vi "DAC Init Results.vi"(8 "error in":errorcluster, 9 "Log Details?":bool, 10 "tdms file":refnum<k34>, 11 "DAC FTCU in":refnum<class "DAC FTCU.lvclass">) -> (0 "error out":errorcluster, 2 "tdms file out":refnum<k34>)   [LabVIEW 2019, in "DAC.lvlib" / "DAC FTCU.lvclass"]
uses:
  DAC FTCU.lvclass
  C:/Users/wg/Documents/LV_Projects/test-stand/App/DAC/DAC.lvclass
  DAC.lvclass/DAC.ctl
  DAC FTCU.lvclass/DAC FTCU.ctl
  DAC.lvclass
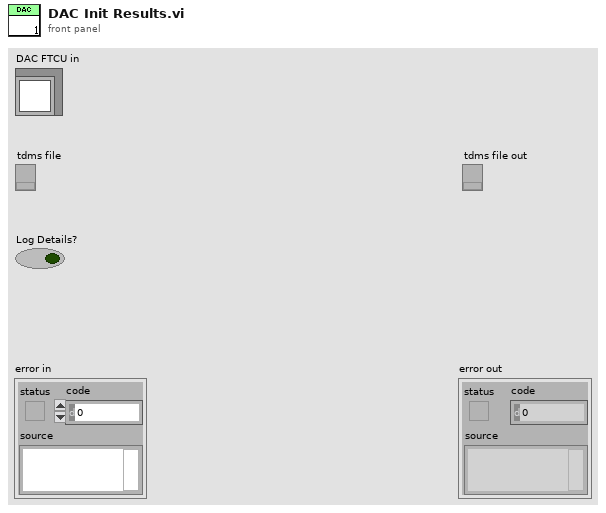
[diagram p1: front panel]
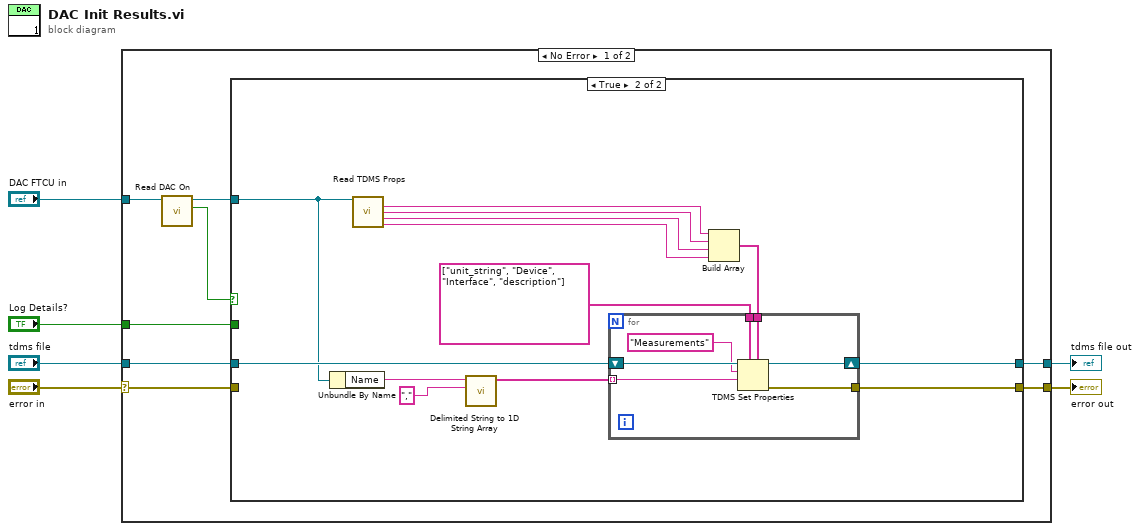
[diagram p0: block diagram]
diagram:
  n1 = case shown="No Error" "error in" {
    selector: "error in" -> [w9 w38]
    tunnel: [w12 w38] -> w3
    tunnel: "DAC FTCU in" -> [w11 _]
    tunnel: "tdms file" -> [w14 w37]
    tunnel: [w13 w37] -> w2
    tunnel: "Log Details?" -> [w7 _]
    frame No Error {
      n2 = call "Read DAC On.vi"("DAC in"=w11) -> ("DAC On"=w8:bool, "DAC out"=w10:refnum<class "DAC FTCU.lvclass">)  [unwired: 8 in, 1 out]
      n3 = case shown="True" w8 {
        tunnel: w14 -> [w16 w29]
        tunnel: [w16 w28] -> w13
        tunnel: [w15 w27] -> w12
        tunnel: w10 -> [_ w26]
        tunnel: w9 -> [w15 _]
        tunnel: w7 -> [_ _]
        frame False {
        }
        frame True {
          n4 = Unbundle By Name(w26) -> ("Name"=w23:string)
          n5 = call "Read TDMS Props.vi"("DAC in"=w26) -> ("Result Unit"=w20:string, "DAC Device"=w19:string, "DAC IO"=w18:string, "DAC Description"=w17:string)  [unwired: 10 in, 1 out]
          n6 = call <vilib>:"Delimited String to 1D String Array.vi"("delimiter"=",", "delimited string"=w23) -> ("string array"=w25:string[])  [unwired: 9 in]
          n7 = Build Array(w20, w19, w18, w17) -> (w22:string[])
          n8 = for {
            tunnel: w25 -> [w34] mode=indexing
            tunnel: string[] ["unit_string", "Device", "Interface", "description"] ("property names") -> [w33]
            tunnel: w22 -> [w32]
            tunnel: [w30] -> w27
            shift-right: [w31] -> w28
            shift-left: w29 -> [w36]
            n9 = TDMS Set Properties(5:w32, 7:w33, 9:w34, 10:"Measurements" ("group name in (Untitled)"), 11:w36) -> (0:w30:errorcluster, 3:w31:refnum<k34>)  [unwired: 1 in, 2 out]
          }
        }
      }
    }
    frame Error {
    }
  }
  "error out" <- w3
  "tdms file out" <- w2
